vi "Configure Stream.vi"(0 "niUsrpRio Session":T1={"FPGA Interface"=refnum, "RIO Interface Number"=0, "Data Clock Rate"=0, "FPGA Data Clock Rate"=0, "Global Settings Register Bus"=refnum, "Radio 0 Settings Register Bus"=refnum, "Radio 1 Settings Register Bus"=refnum, "Radio Settings Bus Semaphore"=refnum, "DB Queues"=[], "Characterization Data Valid?"=FALSE, "EEPROM Header"={"Checksum"=0, "Product Code"=0, "Hardware Current Version"=0, "Hardware Oldest Compatible Version"=0, "EEPROM Map Current Version"=0, "EEPROM Map Oldest Compatible Version"=0, "User Password"="", "Pointer to Factory Header"=0, "Pointer to User Header"=0, "Recommended Interval"=0, "Number of Reserved Bytes"=9, "Number of Daughterboards"=0, "Daughterboard IDs"=[], "Daughterboard Serial Numbers"=[]}, "Device Data Header"={"Checksum"=0, "Number of Channels"=0, "Number of Gain Settings"=[], "Pointer to Characterization Data"=[], "Number of Reserved Bytes"=27, "Number of Frequencies"=[]}, "EEPROM Characterization Header"={"Checksum"=0, "Date"=timestamp(0 s since 1904-01-01), "Temperature"=0.0, "Misc. Info"="", "Pointer to Device Data Header"=0, "Number of Reserved Bytes"=28}, "Characterization Data"=[], "FPGA Current Version"=0, "FPGA Oldest Compatible Version"=0, "Fixed Logic Current Version"=0, "Fixed Logic Oldest Compatible Version"=0, "FPGA Radio Settings Bus Current Version"=0, "FPGA Radio Settings Bus Oldest Compatible Version"=0, "FPGA Board Config Current Version"=0, "FPGA Board Config Oldest Compatible Version"=0} {"FPGA Data Clock Rate" format="%#.3pHz"; "Data Clock Rate" format="%#.3pHz"; "Characterization Data"."Frequencies [Hz]" format="%#_6p"; "EEPROM Characterization Header"."Pointer to Device Data Header" format="%x"; "EEPROM Characterization Header"."Checksum" format="%x"; "Device Data Header"."Pointer to Characterization Data" format="%x"; "Device Data Header"."Checksum" format="%x"; "EEPROM Header"."Pointer to User Header" format="%x"; "EEPROM Header"."Pointer to Factory Header" format="%x"; "EEPROM Header"."Product Code" format="%x"; "EEPROM Header"."Checksum" format="%x"}, 1 "scope":string(combo)="rx", 5 "host FIFO depth":u32=1000000 format="%.0p", 7 "number of samples is finite":bool caption="Number of Samples is Finite", 9 "number of samples":u32=8192 caption="Number of Samples", 11 "error in":errorcluster) -> (4 "niUsrpRio Session (out)":T1={"FPGA Interface"=refnum, "RIO Interface Number"=0, "Data Clock Rate"=0, "FPGA Data Clock Rate"=0, "Global Settings Register Bus"=refnum, "Radio 0 Settings Register Bus"=refnum, "Radio 1 Settings Register Bus"=refnum, "Radio Settings Bus Semaphore"=refnum, "DB Queues"=[], "Characterization Data Valid?"=FALSE, "EEPROM Header"={"Checksum"=0, "Product Code"=0, "Hardware Current Version"=0, "Hardware Oldest Compatible Version"=0, "EEPROM Map Current Version"=0, "EEPROM Map Oldest Compatible Version"=0, "User Password"="", "Pointer to Factory Header"=0, "Pointer to User Header"=0, "Recommended Interval"=0, "Number of Reserved Bytes"=9, "Number of Daughterboards"=0, "Daughterboard IDs"=[], "Daughterboard Serial Numbers"=[]}, "Device Data Header"={"Checksum"=0, "Number of Channels"=0, "Number of Gain Settings"=[], "Pointer to Characterization Data"=[], "Number of Reserved Bytes"=27, "Number of Frequencies"=[]}, "EEPROM Characterization Header"={"Checksum"=0, "Date"=timestamp(0 s since 1904-01-01), "Temperature"=0.0, "Misc. Info"="", "Pointer to Device Data Header"=0, "Number of Reserved Bytes"=28}, "Characterization Data"=[], "FPGA Current Version"=0, "FPGA Oldest Compatible Version"=0, "Fixed Logic Current Version"=0, "Fixed Logic Oldest Compatible Version"=0, "FPGA Radio Settings Bus Current Version"=0, "FPGA Radio Settings Bus Oldest Compatible Version"=0, "FPGA Board Config Current Version"=0, "FPGA Board Config Oldest Compatible Version"=0} {"FPGA Data Clock Rate" format="%#.3pHz"; "Data Clock Rate" format="%#.3pHz"; "Characterization Data"."Frequencies [Hz]" format="%#_6p"; "EEPROM Characterization Header"."Pointer to Device Data Header" format="%x"; "EEPROM Characterization Header"."Checksum" format="%x"; "Device Data Header"."Pointer to Characterization Data" format="%x"; "Device Data Header"."Checksum" format="%x"; "EEPROM Header"."Pointer to User Header" format="%x"; "EEPROM Header"."Pointer to Factory Header" format="%x"; "EEPROM Header"."Product Code" format="%x"; "EEPROM Header"."Checksum" format="%x"}, 15 "error out":errorcluster)   [LabVIEW 2015]
doc: "Configures the stream. This includes configuring the DMA FIFO and the Rx/Tx stream size (in samples).\n\n<B>Input Parameters</B>\n\n<B>host FIFO depth</B> is the number of samples of buffering to request on the host. This value is optional and defaults to eight times the 'number of samples'.\n\n<B>number of samples is finite</B> is used to flag whether this is a continuous acquisition/generation or a finite acquisition/generation.\n\n<B>number of samples</B> to acquire/generate."
uses:
  <instrlib>/niUsrpRio/Config/v1/Host/Public/niUsrpRio Session.ctl
  <instrlib>/_niInstr/Register Bus/v0/Host/Public/Register Bus Session.ctl
  <instrlib>/_niInstr/Register Bus/v0/Host/Private/Session Data.ctl
  <instrlib>/niUsrpRio/Config/v1/Host/Private/DB Queue Reference.ctl
  <instrlib>/niUsrpRio/Config/v1/Host/Private/Daughterboard Data.ctl
  <instrlib>/niUsrpRio/Config/v1/Host/Private/ATR state data.ctl
  <instrlib>/niUsrpRio/Config/v1/Host/Public/EEPROM Header.ctl
  <instrlib>/niUsrpRio/Config/v1/Host/Public/EEPROM Device Data Header.ctl
  <instrlib>/niUsrpRio/Config/v1/Host/Public/EEPROM Characterization Header.ctl
  <instrlib>/niUsrpRio/Config/v1/Host/Public/Characterization Data.ctl
  <instrlib>/niUsrpRio/Config/v1/Host/Public/IQ Imbalance.ctl
  Streaming Xvcr FPGA Ref.ctl
  <vilib>/Utility/error.llb/Error Cluster From Error Code.vi
  <vilib>/rvi/interface/common/niFpgaWaitOnOcc.vi
  <vilib>/rvi/errors/niLvFpgaAdjustHostInterfaceError.vi
  <vilib>/ErrorRing/Error Ring.xnode
  <vilib>/rvi/interface/nirviMethod/nirviMethod.xnode
  <vilib>/rvi/interface/nirviReadWriteControl/nirviReadWriteControl.xnode
  <vilib>/rvi/errors/niLvFpgaMergeErrorWithErrorCode.vi
  <vilib>/rvi/interface/Simulation/niFpgaSimulationCallBeginRW.vi
  NiFpgaLv.dll
  <vilib>/FPGAPlugInAG/Dynamic/niLvFpga_StartFifo_Dynamic.vi
  <vilib>/FPGAPlugInAG/Dynamic/niLvFpga_StopFifo_Dynamic.vi
  <vilib>/FPGAPlugInAG/Dynamic/niLvFpga_ConfigureFifo_Dynamic.vi
  <instrlib>/niUsrpRio/Config/v1/Host/niUsrpRio Config v1 Host.lvlib
  <instrlib>/_niInstr/Register Bus/v0/Host/niInstr Register Bus v0 Host.lvlib
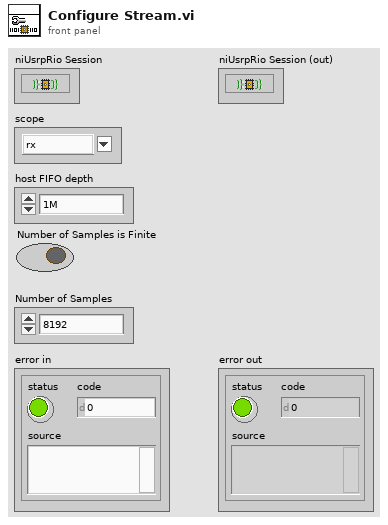
[diagram p1: front panel]
types:
  T1 = typedef "niUsrpRio Config v1 Host.lvlib/niUsrpRio Session.ctl" = cluster{"FPGA Interface":refnum<k20>, "RIO Interface Number":u32, "Data Clock Rate":u32, "FPGA Data Clock Rate":u32, "Global Settings Register Bus":T2, "Radio 0 Settings Register Bus":T2, "Radio 1 Settings Register Bus":T2, "Radio Settings Bus Semaphore":T3, "DB Queues":T4[], "Characterization Data Valid?":bool, "EEPROM Header":T5, "Device Data Header":T6, "EEPROM Characterization Header":T7, "Characterization Data":T8[], "FPGA Current Version":u32, "FPGA Oldest Compatible Version":u32, "Fixed Logic Current Version":u32, "Fixed Logic Oldest Compatible Version":u32, "FPGA Radio Settings Bus Current Version":u32, "FPGA Radio Settings Bus Oldest Compatible Version":u32, "FPGA Board Config Current Version":u32, "FPGA Board Config Oldest Compatible Version":u32}
  T2 = typedef "niInstr Register Bus v0 Host.lvlib/Register Bus Session.ctl" = refnum<queue>
  T3 = typedef "Semaphore RefNum" = refnum<k1>
  T4 = typedef "niUsrpRio Config v1 Host.lvlib/DB Queue Reference.ctl" = refnum<queue>
  T5 = typedef "niUsrpRio Config v1 Host.lvlib/EEPROM Header.ctl" = cluster{"Checksum":u32, "Product Code":u16, "Hardware Current Version":u16, "Hardware Oldest Compatible Version":u16, "EEPROM Map Current Version":u16, "EEPROM Map Oldest Compatible Version":u16, "User Password":string, "Pointer to Factory Header":u32, "Pointer to User Header":u32, "Recommended Interval":u16, "Number of Reserved Bytes":i32, "Number of Daughterboards":u8, "Daughterboard IDs":u16[], "Daughterboard Serial Numbers":string[]}
  T6 = typedef "niUsrpRio Config v1 Host.lvlib/EEPROM Device Data Header.ctl" = cluster{"Checksum":u32, "Number of Channels":u8, "Number of Gain Settings":u16[], "Pointer to Characterization Data":u32[], "Number of Reserved Bytes":i32, "Number of Frequencies":u16[]}
  T7 = typedef "niUsrpRio Config v1 Host.lvlib/EEPROM Characterization Header.ctl" = cluster{"Checksum":u32, "Date":timestamp, "Temperature":sgl, "Misc. Info":string, "Pointer to Device Data Header":u32, "Number of Reserved Bytes":i32}
  T8 = typedef "niUsrpRio Config v1 Host.lvlib/Characterization Data.ctl" = cluster{"Gains[dB]":dbl[], "Frequencies [Hz]":dbl[], "IQ Imbalance Table":T9[], "Measured Gains[dB]":dbl[][]}
  T9 = typedef "niUsrpRio Config v1 Host.lvlib/IQ Imbalance.ctl" = cluster{"Gain Imbalance [linear]":dbl, "Phase Imbalance [radians]":dbl, "Offset":cdb}
  T10 = typedef "Streaming Xvcr FPGA Ref.ctl" = refnum<k20>
  T11 = typedef "niUsrpRio Config v1 Host.lvlib/Device Subfunction.ctl" = enum16{"rx", "tx", "all"}
  T12 = typedef "niUsrpRio Config v1 Host.lvlib/RF Channel.ctl" = enum16{"0", "1", "All"}
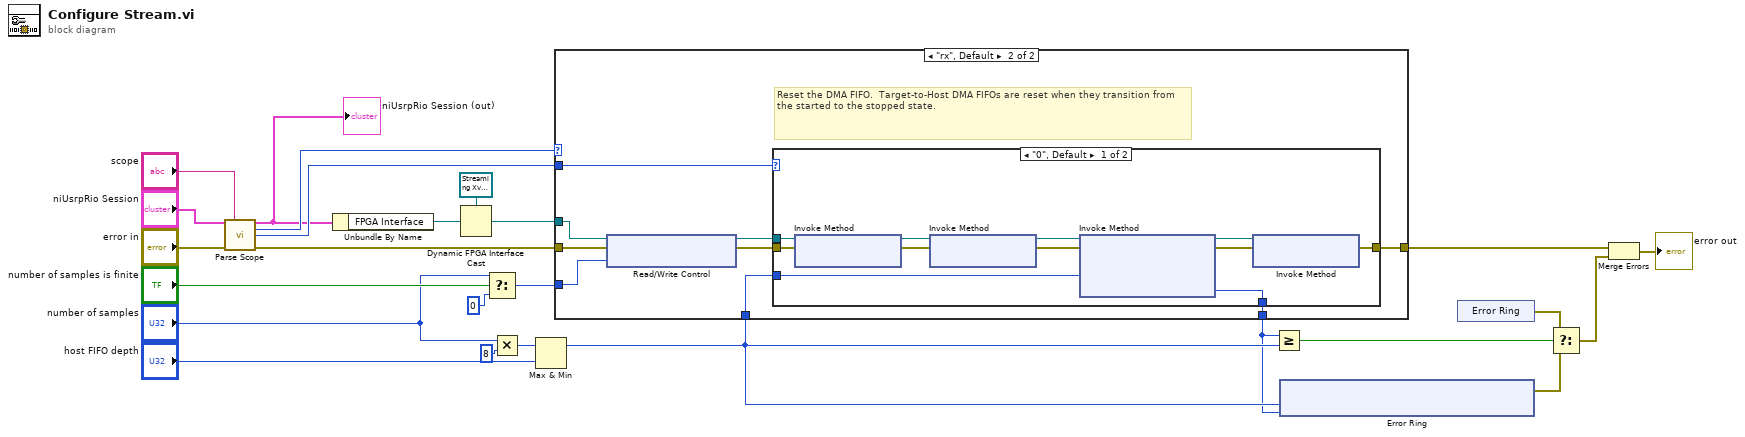
[diagram p0: block diagram]
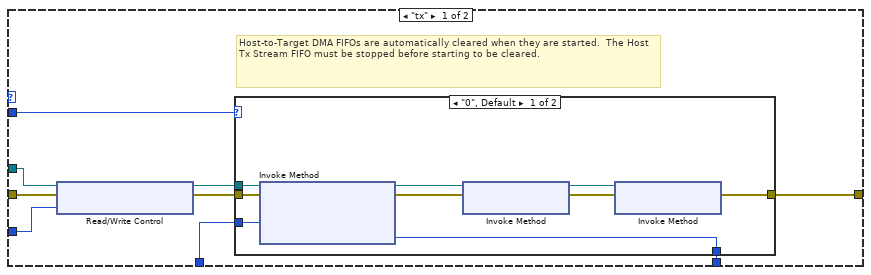
[diagram p2: hidden frame]
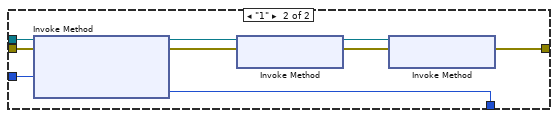
[diagram p3: hidden frame]
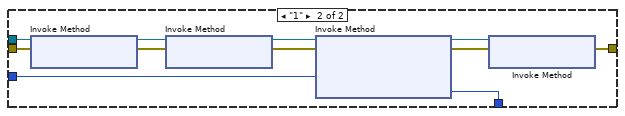
[diagram p4: hidden frame]
diagram:
  n1 = call <instrlib>:"Parse Scope.vi"("niUsrpRio Session"="niUsrpRio Session", "scope"="scope", "error in"="error in") -> ("niUsrpRio Session (out)"=w8:T1, "Device Subfunction"=w10:T11, "Device Subfunction Channel"=w9:T12, "error out"=w7:errorcluster)  [unwired: 4 in, 5 out]
  "niUsrpRio Session (out)" <- w8
  n2 = Unbundle By Name(w8) -> ("FPGA Interface"=w3:refnum<k20>)
  n3 = Dynamic FPGA Interface Cast(Session In=T10 refnum ("Type"), Type=w3) -> (Session Out=w2:T10)
  n4 = Select(t="number of samples", s="number of samples is finite", f=u32 0) -> (s? t:f=w19:u32)
  n5 = Multiply(x="number of samples", y=u32 8 ("x")) -> (x*y=w24:u32)
  n6 = Max & Min(x=w24, y="host FIFO depth") -> (max(x,y)=w12:u32)  [unwired: 1 out]
  n7 = case shown="\"rx\", Default" w10 {
    tunnel: w12 -> [w31 w60]
    tunnel: [w34 w61] -> w15
    tunnel: w19 -> [w30 w59]
    tunnel: [w29 w56] -> w11
    tunnel: w7 -> [w28 w55]
    tunnel: w9 -> [w27 w54]
    tunnel: w2 -> [w26 w53]
    frame "tx" {
      # "Host-to-Target DMA FIFOs are automatically cleared when they are started.  The Host Tx Stream FIFO must be stopped before starting to be cleared."
      n8 = xnode "Read/Write Control"("FPGA VI Reference In"=w26, "error in"=w28, "tx.samples to generate"=w30) -> ("FPGA VI Reference Out"=w32:T10, "error out"=w33:errorcluster)
      n9 = case shown="\"0\", Default" w27 {
        tunnel: [w43 w44] -> w34
        tunnel: w33 -> [w42 w47]
        tunnel: w32 -> [w41 w48]
        tunnel: w31 -> [w36 w46]
        tunnel: [w35 w45] -> w29
        frame "0", Default {
          n10 = xnode "Invoke Method"("FPGA VI Reference In"=w41, "error in"=w42, "Requested Depth"=w36) -> ("FPGA VI Reference Out"=w39:T10, "error out"=w40:errorcluster, "Actual Depth"=w35:u32)
          n11 = xnode "Invoke Method"("FPGA VI Reference In"=w39, "error in"=w40) -> ("FPGA VI Reference Out"=w37:T10, "error out"=w38:errorcluster)
          n12 = xnode "Invoke Method"("FPGA VI Reference In"=w37, "error in"=w38) -> ("error out"=w43:errorcluster)  [unwired: 1 out]
        }
        frame "1" {
          n13 = xnode "Invoke Method"("FPGA VI Reference In"=w48, "error in"=w47, "Requested Depth"=w46) -> ("FPGA VI Reference Out"=w51:T10, "error out"=w52:errorcluster, "Actual Depth"=w45:u32)
          n14 = xnode "Invoke Method"("FPGA VI Reference In"=w51, "error in"=w52) -> ("FPGA VI Reference Out"=w49:T10, "error out"=w50:errorcluster)
          n15 = xnode "Invoke Method"("FPGA VI Reference In"=w49, "error in"=w50) -> ("error out"=w44:errorcluster)  [unwired: 1 out]
        }
      }
    }
    frame "rx", Default {
      # "Reset the DMA FIFO.  Target-to-Host DMA FIFOs are reset when they transition from the started to the stopped state."
      n16 = xnode "Read/Write Control"("FPGA VI Reference In"=w53, "error in"=w55, "rx.samples to acquire"=w59) -> ("FPGA VI Reference Out"=w57:T10, "error out"=w58:errorcluster)
      n17 = case shown="\"0\", Default" w54 {
        tunnel: [w70 w81] -> w61
        tunnel: w60 -> [w65 w76]
        tunnel: w58 -> [w64 w75]
        tunnel: w57 -> [w63 w74]
        tunnel: [w62 w73] -> w56
        frame "0", Default {
          n18 = xnode "Invoke Method"("FPGA VI Reference In"=w63, "error in"=w64) -> ("FPGA VI Reference Out"=w68:T10, "error out"=w69:errorcluster)
          n19 = xnode "Invoke Method"("FPGA VI Reference In"=w68, "error in"=w69) -> ("FPGA VI Reference Out"=w67:T10, "error out"=w66:errorcluster)
          n20 = xnode "Invoke Method"("FPGA VI Reference In"=w67, "error in"=w66, "Requested Depth"=w65) -> ("FPGA VI Reference Out"=w72:T10, "error out"=w71:errorcluster, "Actual Depth"=w62:u32)
          n21 = xnode "Invoke Method"("FPGA VI Reference In"=w72, "error in"=w71) -> ("error out"=w70:errorcluster)  [unwired: 1 out]
        }
        frame "1" {
          n22 = xnode "Invoke Method"("FPGA VI Reference In"=w74, "error in"=w75) -> ("FPGA VI Reference Out"=w79:T10, "error out"=w80:errorcluster)
          n23 = xnode "Invoke Method"("FPGA VI Reference In"=w79, "error in"=w80) -> ("FPGA VI Reference Out"=w78:T10, "error out"=w77:errorcluster)
          n24 = xnode "Invoke Method"("FPGA VI Reference In"=w78, "error in"=w77, "Requested Depth"=w76) -> ("FPGA VI Reference Out"=w83:T10, "error out"=w82:errorcluster, "Actual Depth"=w73:u32)
          n25 = xnode "Invoke Method"("FPGA VI Reference In"=w83, "error in"=w82) -> ("error out"=w81:errorcluster)  [unwired: 1 out]
        }
      }
    }
  }
  n26 = Greater Or Equal?(x=w11, y=w12) -> (x >= y?=w13:bool)
  n27 = xnode ("Error Ring")("parameter 0"=w12, "parameter 1"=w11) -> ("error out"=w17:errorcluster)
  n28 = xnode ("Error Ring")() -> ("error out"=w16:errorcluster)
  n29 = Select(t=w16, s=w13, f=w17) -> (s? t:f=w18:errorcluster)
  n30 = Merge Errors(w15, w18) -> (→"error out":errorcluster)
